vi "Get Position (SubVI).vi"(8 "error in (no error)":errorcluster, 10 "Axis":i32, 11 ".NET Refnum in":refnum<k24>) -> (0 "error out":errorcluster, 2 "position":dbl)   [LabVIEW 2019, in "ESP301.lvlib"]
uses:
  ESP301.lvlib
  Newport.ESP301.CommandInterface
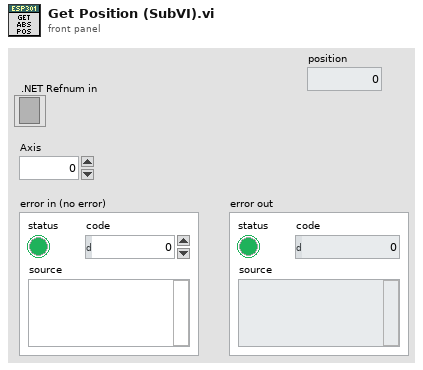
[diagram p1: front panel]
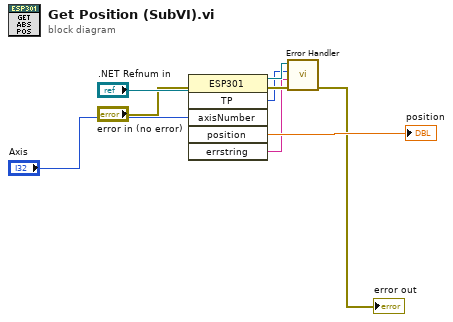
[diagram p0: block diagram]
diagram:
  n1 = invoke class="ESP301" method="TP"(reference=".NET Refnum in", error in="error in (no error)", "axisNumber"="Axis") -> (reference out=w3:refnum<k24>, error out=w7:errorcluster, "TP"=w2:i32, "position"=→"position":dbl, "errstring"=w1:string)  [unwired: 3 in, 1 out]
  n2 = call "Error Handler.vi"("error in (no error)"=w7, "value"=w1, "OpenInstrument"=w2, ".NET Refnum in"=w3) -> ("error out"=→"error out":errorcluster)  [unwired: 6 in, 1 out]
